vi "Setup ILC.vi"(8 "error in (no error)":errorcluster, 10 "Model in":refnum<class "Model.lvclass">, 11 "Boot Loader in":refnum<class "Boot Loader.lvclass">) -> (0 "error out":errorcluster, 2 "Model out":refnum<class "Model.lvclass">, 3 "Boot Loader out":refnum<class "Boot Loader.lvclass">)   [LabVIEW 2016, in "Boot Loader.lvclass"]
uses:
  Boot Loader.lvclass
  Model/Model.lvclass
  Modbus/DesktopModbus/DesktopModbus.lvclass
  Common_RT_FAILC/FAILCFactory/FAILCFactory.lvclass
  Modbus/DesktopModbus/DesktopModbus.lvclass/DesktopModbus.ctl
  Model/Model.lvclass/Model.ctl
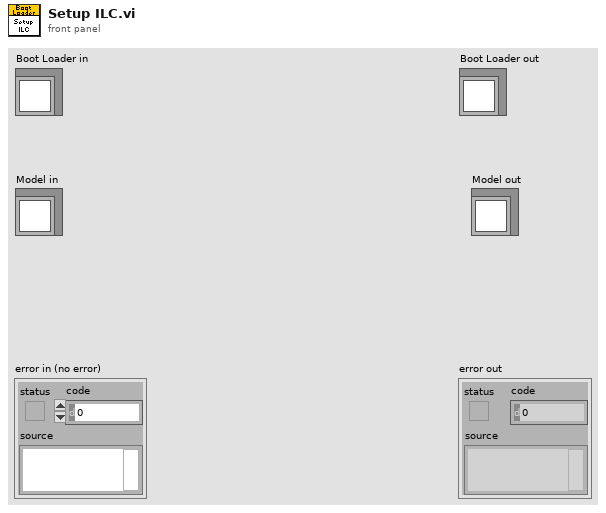
[diagram p1: front panel]
types:
  T1 = typedef "FAMT Typedefs.lvlib/SerialSettings.ctl" = cluster{"Baud Rate":u32, "Data Bits":u16, "Parity":enum16{"None", "Odd", "Even", "Mark", "Space"}, "Flow Control":u16, "Stop Bits":u16, "Timeout (ms)":u32, "Byte Count":u32, "Enable Termination Character":bool, "Termination Char":u8}
  T2 = typedef "RTFAILC.lvlib/FASettings.ctl" = cluster{"ILCSettings":T3, "ID":i16, "FATypes":T4}
  T3 = typedef "RTILC.lvlib/ILCSettings.ctl" = cluster{"Subnet":u8, "Address":u8}
  T4 = typedef "RTFAILC.lvlib/FATypes.ctl" = enum16{"SingleAxis", "LateralDualAxis", "CrossLateralDualAxis"}
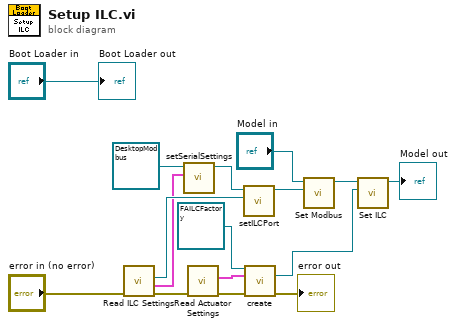
[diagram p0: block diagram]
diagram:
  n1 = call "Read ILC Settings.vi"("error in (no error)"="error in (no error)") -> ("error out"=w3:errorcluster, "Serial Settings"=w10:T1, "ILC Port"=w11:refnum<visa-resource-name>)  [unwired: 7 in, 1 out]
  n2 = call "setSerialSettings.vi"("Serial Settings"=w10, "DesktopModbus in"=refnum<class "DesktopModbus.lvclass"> refnum ("DesktopModbus.lvclass")) -> ("DesktopModbus out"=w12:refnum<class "DesktopModbus.lvclass">)  [unwired: 9 in]
  n3 = call "Read Actuator Settings.vi"("error in (no error)"=w3) -> ("error out"=w5:errorcluster, "FASettings"=w6:T2)  [unwired: 8 in, 1 out]
  n4 = call "setILCPort.vi"("ILC Port"=w11, "DesktopModbus in"=w12) -> ("DesktopModbus out"=w4:refnum<class "DesktopModbus.lvclass">)  [unwired: 9 in]
  n5 = call "create.vi"("FAILCFactory in"=refnum<class "FAILCFactory.lvclass"> refnum ("RTFAILC.lvlib:FAILCFactory.lvclass"), "FASettings"=w6, "error in (no error)"=w5) -> ("ForceActuator"=w7:refnum<class "FAILC.lvclass">, "error out"=→"error out":errorcluster)  [unwired: 10 in, 1 out]
  n6 = call "Set Modbus.vi"("Modbus"=w4, "Model in"="Model in") -> ("Model out"=w9:refnum<class "Model.lvclass">)  [unwired: 9 in]
  n7 = call "Set ILC.vi"("ILC"=w7, "Model in"=w9) -> ("Model out"=→"Model out":refnum<class "Model.lvclass">)  [unwired: 9 in]
  "Boot Loader out" <- "Boot Loader in"
